vi "3.vi"(9 "3":dbl, 10 "Numeric":i32, 11 "Numeric 2":i32) -> (3 "Array":u32[](array[numeric]))   [LabVIEW 2016]
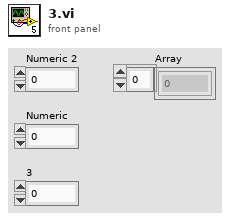
[diagram p1: front panel]
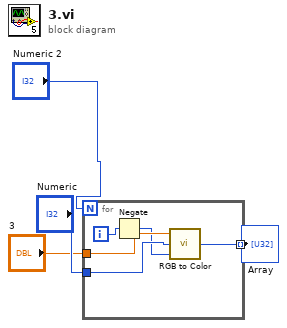
[diagram p0: block diagram]
diagram:
  n1 = for {
    N: "Numeric 2" -> [_]
    tunnel: [w9] -> w4 mode=indexing
    tunnel: "3" -> [w8]
    tunnel: "Numeric" -> [w7]
    i -> [w6]
    n2 = Negate(x=w6) -> (-x=w5:i32)
    n3 = call <vilib>:"RGB to Color.vi"("B"=w5, "G"=w7, "R"=w8) -> ("Color"=w9:u32)
  }
  "Array" <- w4
